vi "ReadBlueSerializableVersionPathWrapper.vi"(8 "error in (no error)":errorcluster, 10 "Application":refnum<vi>, 11 "LVClass name":string) -> (0 "error out":errorcluster, 2 "BlueSerializableVersion found?":bool, 3 "BlueSerializableVersion":u16)   [LabVIEW 2019, in "BlueSerializationScripts.lvlib"]
uses:
  BlueSerializationScripts.lvlib
  UserAppLibs/IncrementMutationHistory/IncrementMutationHistory.lvlib
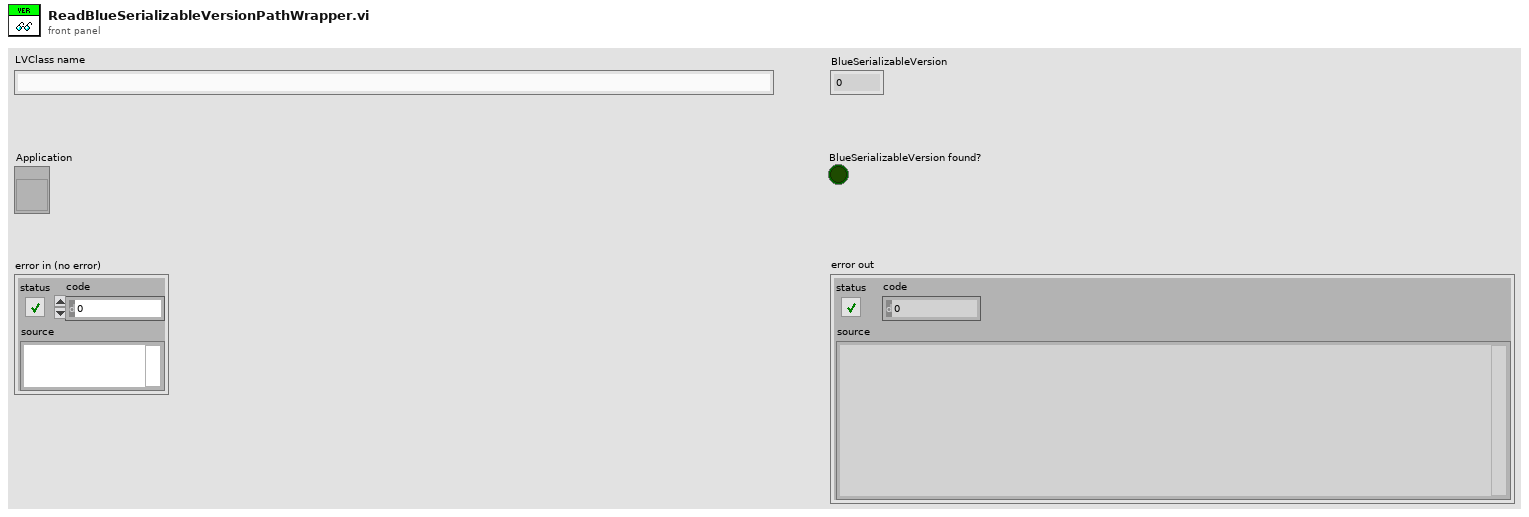
[diagram p1: front panel]
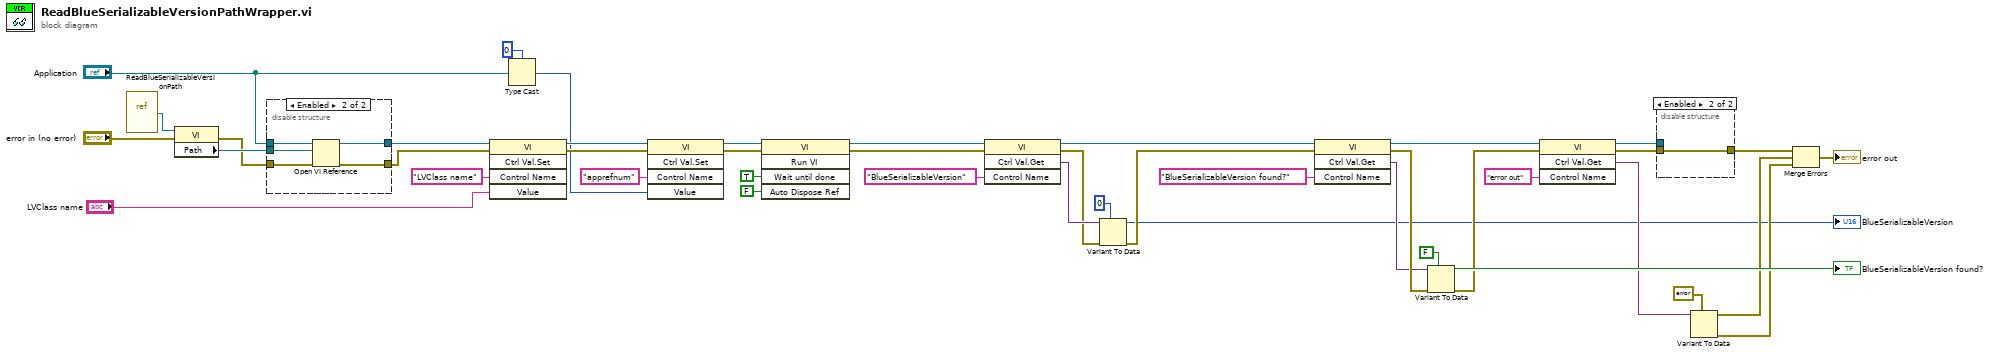
[diagram p0: block diagram]
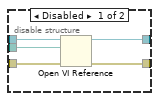
[diagram p2: hidden frame]
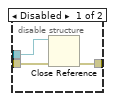
[diagram p3: hidden frame]
diagram:
  n1 = vi-ref "ReadBlueSerializableVersionPath.vi"() -> (w42:refnum<vi>)
  n2 = property class="VI"(reference=w42, error in="error in (no error)") -> (error out=w40:errorcluster, "Path"=w41:path)  [unwired: 1 out]
  n3 = disable-structure shown="Enabled" {
    disable-tunnel: w41 -> [w48 w52]
    disable-tunnel: w40 -> [w47 w53]
    disable-tunnel: [w46 w50] -> w18
    disable-tunnel: [w45 w49] -> w19
    disable-tunnel: "Application" -> [w44 w51]
    frame Disabled {
      n4 = Open VI Reference(application reference (local)=w44, vi path=w48, error in (no error)=w47) -> (vi reference=w46:refnum<vi>, error out=w45:errorcluster)  [unwired: 3 in]
    }
    frame Enabled {
      n5 = Open VI Reference(application reference (local)=w51, vi path=w52, error in (no error)=w53) -> (vi reference=w50:refnum<vi>, error out=w49:errorcluster)  [unwired: 3 in]
    }
  }
  n6 = invoke class="VI" method="Ctrl Val.Set"(reference=w18, error in=w19, "Control Name"="LVClass name", "Value"="LVClass name") -> (reference out=w15:refnum<vi>, error out=w16:errorcluster)  [unwired: 1 in, 3 out]
  n7 = Type Cast(type=u32 0, x="Application") -> (*(type *) &x=w11:u32)
  n8 = invoke class="VI" method="Ctrl Val.Set"(reference=w15, error in=w16, "Control Name"="apprefnum", "Value"=w11) -> (reference out=w13:refnum<vi>, error out=w14:errorcluster)  [unwired: 1 in, 3 out]
  n9 = invoke class="VI" method="Run VI"(reference=w13, error in=w14, "Wait until done"=TRUE ("Wait Until Done"), "Auto Dispose Ref"=FALSE ("Auto Dispose Reference")) -> (reference out=w6:refnum<vi>, error out=w5:errorcluster)  [unwired: 1 in, 3 out]
  n10 = invoke class="VI" method="Ctrl Val.Get"(reference=w6, error in=w5, "Control Name"="BlueSerializableVersion") -> (reference out=w4:refnum<vi>, error out=w8:errorcluster, "Get Control Value Variant"=w9:variant)  [unwired: 1 in, 1 out]
  n11 = Variant To Data(error in=w8, type=u16 0 ("BlueSerializableVersion"), Variant=w9) -> (data=→"BlueSerializableVersion":u16, error out=w3:errorcluster)
  n12 = invoke class="VI" method="Ctrl Val.Get"(reference=w4, error in=w3, "Control Name"="BlueSerializableVersion found?") -> (reference out=w33:refnum<vi>, error out=w32:errorcluster, "Get Control Value Variant"=w31:variant)  [unwired: 1 in, 1 out]
  n13 = Variant To Data(error in=w32, type=FALSE, Variant=w31) -> (data=→"BlueSerializableVersion found?":bool, error out=w28:errorcluster)
  n14 = invoke class="VI" method="Ctrl Val.Get"(reference=w33, error in=w28, "Control Name"="error out") -> (reference out=w20:refnum<vi>, error out=w22:errorcluster, "Get Control Value Variant"=w27:variant)  [unwired: 1 in, 1 out]
  n15 = disable-structure shown="Enabled" {
    disable-tunnel: w22 -> [w56 w57]
    disable-tunnel: [w55 w57] -> w21
    disable-tunnel: w20 -> [w54 _]
    frame Disabled {
      n16 = Close Reference(reference=w54, error in (no error)=w56) -> (error out=w55:errorcluster)
    }
    frame Enabled {
    }
  }
  n17 = Variant To Data(type=errorcluster {"status"=FALSE, "code"=0, "source"=""} ("error out"), Variant=w27) -> (data=w25:errorcluster, error out=w24:errorcluster)  [unwired: 1 in]
  n18 = Merge Errors(w21, w25, w24) -> (→"error out":errorcluster)
